vi "Program Synth.vi"(8 "error in (no error)":errorcluster, 11 "NHMFL Synthesizer in":refnum<class "NHMFL Synthesizer.lvclass">) -> (0 "error out":errorcluster, 3 "NHMFL Synthesizer out":refnum<class "NHMFL Synthesizer.lvclass">)   [LabVIEW 2016, in "NHMFL Synthesizer.lvclass"]
uses:
  NHMFL Synthesizer.lvclass
  C:/Program Files/National Instruments/LabVIEW 2016/vi.lib/ActorFramework/Actor/Actor.lvclass
  <vilib>/ActorFramework/Actor/Actor.lvclass/Actor.ctl
  NHMFL Synthesizer.lvclass/NHMFL Synthesizer.ctl
  Template Module Messages/Write FP Control Msg/Write FP Control Msg.lvclass
  C:/Program Files/National Instruments/LabVIEW 2016/vi.lib/ActorFramework/Message/Message.lvclass
  Template Module Messages/Write FP Control Msg/Write FP Control Msg.lvclass/Write FP Control Msg.ctl
  Template Module Messages/Message Nested Object Msg/Message Nested Object Msg.lvclass/Message Nested Object Msg.ctl
  <vilib>/ActorFramework/Message Enqueuer/Message Enqueuer.lvclass/Message Enqueuer.ctl
  Template Module Messages/Write FP Control Msg/Write Field name.vi
  Template Module Messages/Write FP Control Msg/Write Control Name.vi
  Template Module Messages/Write FP Control Msg/Write Control Value.vi
  <vilib>/ActorFramework/Message Enqueuer/Enqueue.vi
  Template Module Messages/Message Nested Object Msg/Message Nested Object Msg.lvclass
  Read NHMFL Synthesizer Configuration.vi
  <vilib>/ActorFramework/Message Priority Queue/Priority Enqueue.vi
  <vilib>/ActorFramework/Actor/Actor.lvclass
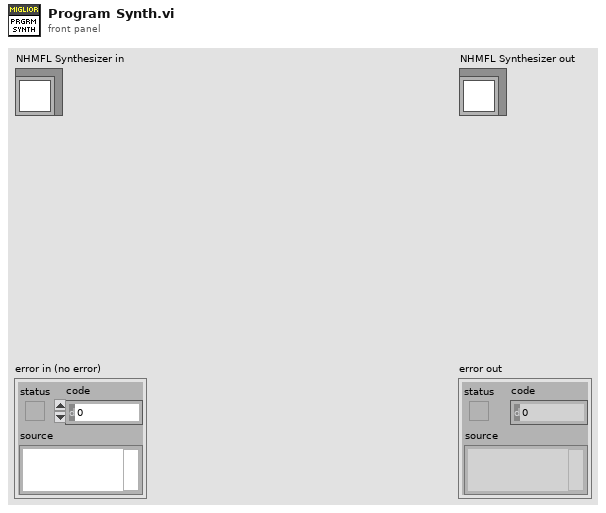
[diagram p1: front panel]
types:
  T1 = typedef "NHMFL Synthesizer Configuration.ctl" = cluster{"DAQmx Device":tag, "Variable amplitude frequency":dbl, "Fixed amplitude frequency":dbl, "Amplitude":dbl, "Clock multiplier":i32, "Channel names (variable F)":string[], "Channel names (fixed F)":string[], "Group":string, "Auto-update other modules":bool, "Recorder module":string, "Lock-in module ":string}
  T2 = typedef "Lockin Parameters.ctl" = cluster{"Frequency":dbl, "Phase":dbl, "Syncronous":bool, "Points per sine wave":i32, "DDS":bool, "Frequency word":u32, "Phase word":u32, "DDS modulus":i64, "DDS clock":dbl}
  T3 = typedef "Actual settings.ctl" = cluster{"Clock/F1":ext, "Clock/F2":ext, "F1":ext, "F2":ext, "Clock":ext}
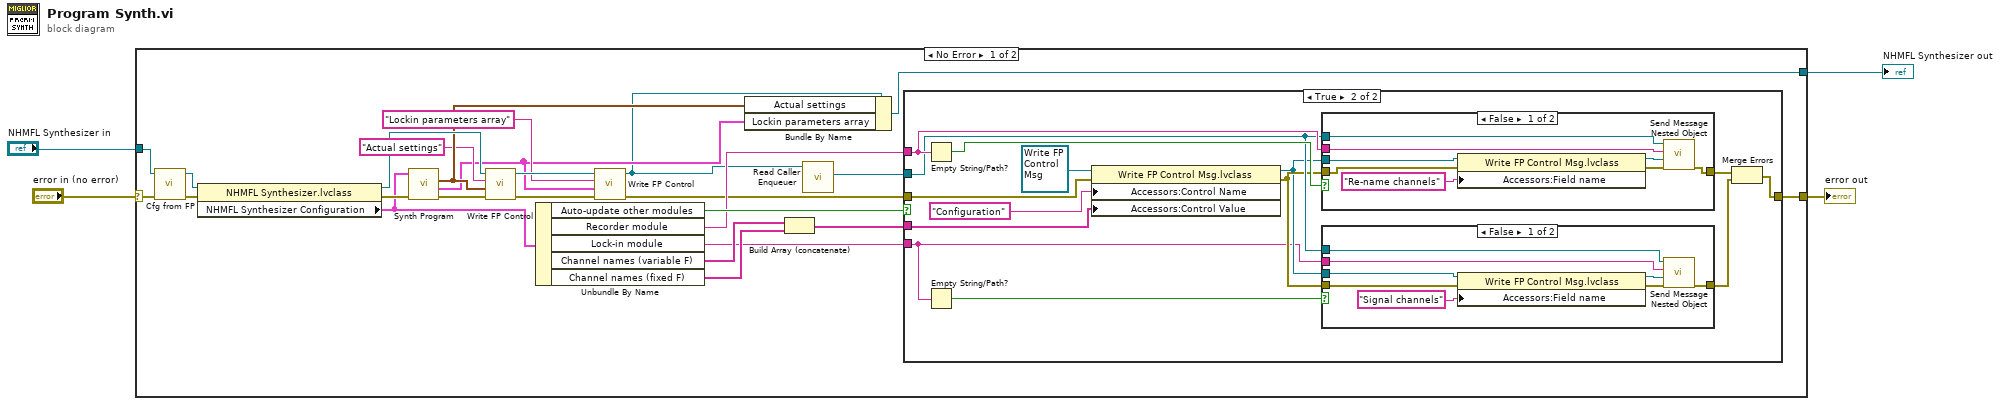
[diagram p0: block diagram]
diagram:
  n1 = case shown="No Error" "error in (no error)" {
    selector: "error in (no error)" -> [w23 w64]
    tunnel: [w5 w64] -> w3
    tunnel: [w28 w63] -> w1
    tunnel: "NHMFL Synthesizer in" -> [w20 w63]
    frame No Error {
      n2 = call-dynamic "Cfg from FP.vi"("error in (no error)"=w23, "Measure Object in"=w20) -> ("error out"=w22:errorcluster, "Measure Object out"=w29:refnum<class "NHMFL Synthesizer.lvclass">)  [unwired: 8 in]
      n3 = property class="NHMFL Synthesizer.lvclass"(reference=w29, error in=w22) -> (reference out=w26:refnum<class "NHMFL Synthesizer.lvclass">, error out=w27:errorcluster, "NHMFL Synthesizer Configuration"=w15:T1)
      n4 = call "Synth Program.vi"("Error In"=w27, "User configuration"=w15) -> ("Error Out"=w21:errorcluster, "Lockin parameters array"=w16:T2[], "Actual ratios"=w25:T3)  [unwired: 6 in, 1 out]
      n5 = call-dynamic "Write FP Control.vi"("error in (no error)"=w21, "Control Value"=w25, "Control Name"="Actual settings", "Measure Object in"=w26) -> ("error out"=w18:errorcluster, "Measure Object out"=w19:refnum<class "NHMFL Synthesizer.lvclass">)  [unwired: 6 in]
      n6 = Unbundle By Name(w15) -> ("Auto-update other modules"=w14:bool, "Recorder module"=w13:string, "Lock-in module"=w6:string, "Channel names (variable F)"=w9:string[], "Channel names (fixed F)"=w8:string[])
      n7 = call-dynamic "Write FP Control.vi"("error in (no error)"=w18, "Control Value"=w16, "Control Name"="Lockin parameters array", "Measure Object in"=w19) -> ("error out"=w10:errorcluster, "Measure Object out"=w12:refnum<class "NHMFL Synthesizer.lvclass">)  [unwired: 6 in]
      n8 = Bundle By Name(cluster=w12, "Actual settings"=w25, "Lockin parameters array"=w16) -> (w28:refnum<class "NHMFL Synthesizer.lvclass">)
      n9 = Build Array (concatenate)(w9, w8) -> (w7:string[])
      n10 = call <vilib>:"Read Caller Enqueuer.vi"("Actor"=w12) -> ("Caller Enqueuer"=w11:refnum<class "Message Enqueuer.lvclass">)  [unwired: 10 in]
      n11 = case shown="True" w14 {
        tunnel: w13 -> [_ w43]
        tunnel: w11 -> [_ w37]
        tunnel: w10 -> [w30 w41]
        tunnel: w7 -> [_ w39]
        tunnel: w6 -> [_ w34]
        tunnel: [w30 w31] -> w5
        frame False {
        }
        frame True {
          n12 = Empty String/Path?(string/path=w43) -> (empty?=w44:bool)
          n13 = Empty String/Path?(string/path=w34) -> (empty?=w38:bool)
          n14 = property class="Write FP Control Msg.lvclass"(reference=refnum<class "Write FP Control Msg.lvclass"> refnum ("Write FP Control Msg.lvclass"), error in=w41, "Accessors:Control Name"="Configuration", "Accessors:Control Value"=w39) -> (reference out=w35:refnum<class "Write FP Control Msg.lvclass">, error out=w36:errorcluster)
          n15 = case shown="False" w44 {
            tunnel: w37 -> [w61 _]
            tunnel: w43 -> [w60 _]
            tunnel: w36 -> [w58 w62]
            tunnel: w35 -> [w59 _]
            tunnel: [w54 w62] -> w33
            frame False {
              n16 = property class="Write FP Control Msg.lvclass"(reference=w59, error in=w58, "Accessors:Field name"="Re-name channels" ("Field name")) -> (reference out=w56:refnum<class "Write FP Control Msg.lvclass">, error out=w55:errorcluster)
              n17 = call "Send Message Nested Object.vi"("error in (no error)"=w55, "Message"=w56, "Name"=w60, "Message Enqueuer"=w61) -> ("error out"=w54:errorcluster)  [unwired: 6 in, 1 out]
            }
            frame True {
            }
          }
          n18 = case shown="False" w38 {
            tunnel: w37 -> [w52 _]
            tunnel: w34 -> [w51 _]
            tunnel: w36 -> [w49 w53]
            tunnel: w35 -> [w50 _]
            tunnel: [w45 w53] -> w32
            frame False {
              n19 = property class="Write FP Control Msg.lvclass"(reference=w50, error in=w49, "Accessors:Field name"="Signal channels" ("Field name")) -> (reference out=w47:refnum<class "Write FP Control Msg.lvclass">, error out=w46:errorcluster)
              n20 = call "Send Message Nested Object.vi"("error in (no error)"=w46, "Message"=w47, "Name"=w51, "Message Enqueuer"=w52) -> ("error out"=w45:errorcluster)  [unwired: 6 in, 1 out]
            }
            frame True {
            }
          }
          n21 = Merge Errors(w33, w32) -> (w31:errorcluster)
        }
      }
    }
    frame Error {
    }
  }
  "error out" <- w3
  "NHMFL Synthesizer out" <- w1
